vi "Get All Status Channels.vi"(8 "error in (no error)":errorcluster, 11 "VeriStand Data Sharing Framework in":refnum<class "VeriStand DSF.lvclass">) -> (0 "error out":errorcluster, 2 "status channel offsets":u64[](array[numeric]) format="%.0x", 3 "VeriStand Data Sharing Framework out":refnum<class "VeriStand DSF.lvclass">)   [LabVIEW 2017, in "DSF Engine.lvlib" / "VeriStand DSF.lvclass"]
uses:
  VeriStand DSF.lvclass
  VeriStand DSF.lvclass/VeriStand DSF.ctl
  <vilib>/NI Veristand/Custom Device API/Data Access Type.ctl
  <vilib>/NI Veristand/Custom Device API/Custom Device API.lvlib
  Shared/DSF Shared.lvlib
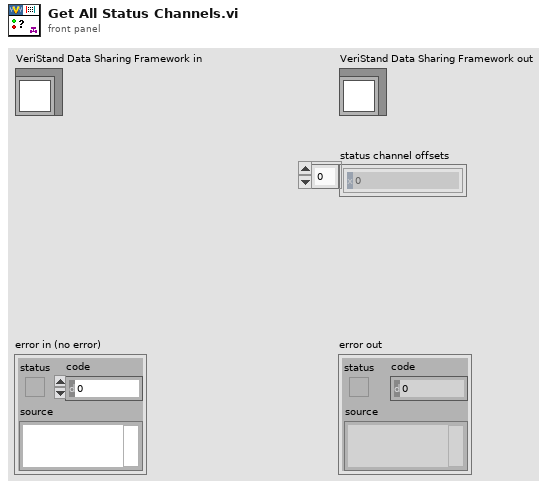
[diagram p1: front panel]
types:
  T1 = enum16{"open", "replace", "create", "open or create", "replace or create", "replace or create with confirmation"}
  T2 = typedef "Custom Device API.lvlib/Custom Device Item Ref.ctl" = u64
  T3 = typedef "Custom Device API.lvlib/Data Access Type.ctl" = enum16{"Read", "Write"}
  T4 = typedef "Custom Device API.lvlib/Data Reference.ctl" = i32
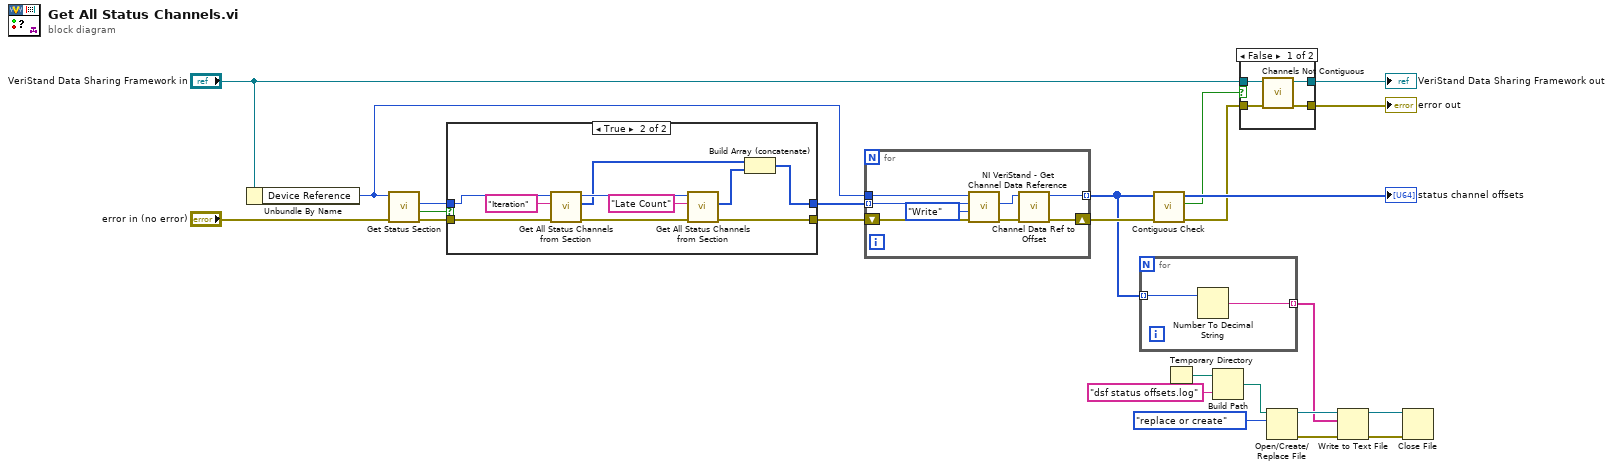
[diagram p0: block diagram]
diagram:
  n1 = Unbundle By Name("VeriStand Data Sharing Framework in") -> ("Device Reference"=w9:T2)
  n2 = call "Get Status Section.vi"("error in (no error)"="error in (no error)", "Item Ref in"=w9) -> ("error out"=w14:errorcluster, "found"=w2:bool, "Status Section ref"=w13:T2)  [unwired: 6 in, 1 out]
  n3 = case shown="True" w2 {
    tunnel: w14 -> [w25 w34]
    tunnel: w13 -> [_ w33]
    tunnel: [w25 w26] -> w12
    tunnel: [_ w35] -> w1
    frame False {
    }
    frame True {
      n4 = call "Get All Status Channels from Section.vi"("error in (no error)"=w34, "Section Name"="Iteration", "Item Ref in"=w33) -> ("error out"=w30:errorcluster, "status channels refs"=w28:T2[], "Item Ref out"=w31:T2)  [unwired: 6 in]
      n5 = call "Get All Status Channels from Section.vi"("error in (no error)"=w30, "Section Name"="Late Count", "Item Ref in"=w31) -> ("error out"=w26:errorcluster, "status channels refs"=w27:T2[])  [unwired: 6 in, 1 out]
      n6 = Build Array (concatenate)(w28, w27) -> (w35:T2[])
    }
  }
  n7 = for {
    shift-right: [w42] -> w11
    shift-left: w12 -> [w41]
    tunnel: [w39] -> w10 mode=indexing
    tunnel: w9 -> [w37]
    tunnel: w1 -> [w36] mode=indexing
    n8 = call <vilib>:"NI VeriStand - Get Channel Data Reference.vi"("error in (no error)"=w41, "Access"=Data_Access_Type."Write", "Channel Ref in"=w36, "Device Ref in"=w37) -> ("error out"=w43:errorcluster, "Channel Data Reference"=w40:T4)  [unwired: 5 in, 1 out]
    n9 = call "Channel Data Ref to Offset.vi"("error in (no error)"=w43, "Channel Data Reference"=w40) -> ("error out"=w42:errorcluster, "channel offset"=w39:u64)  [unwired: 8 in]
  }
  n10 = for {
    tunnel: [w45] -> w16 mode=indexing
    tunnel: w10 -> [w44] mode=indexing
    n11 = Number To Decimal String(number=w44) -> (decimal integer string=w45:string)  [unwired: 1 in]
  }
  n12 = call "Contiguous Check.vi"("error in (no error)"=w11, "channel offsets in"=w10) -> ("error out"=w4:errorcluster, "contiguous?"=w3:bool, "channel offsets out"=→"status channel offsets":u64[])  [unwired: 7 in]
  n13 = Temporary Directory() -> (w23:path)
  n14 = Build Path(base path=w23, name or relative path="dsf status offsets.log") -> (appended path=w21:path)
  n15 = case shown="False" w3 {
    tunnel: "VeriStand Data Sharing Framework in" -> [w49 w51]
    tunnel: [w48 w51] -> w7
    tunnel: [w47 w50] -> w6
    tunnel: w4 -> [w46 w50]
    frame False {
      n16 = call "Channels Not Contiguous.vi"("error in (no error)"=w46, "VeriStand DSF in"=w49) -> ("error out"=w47:errorcluster, "VeriStand DSF out"=w48:refnum<class "VeriStand DSF.lvclass">)  [unwired: 8 in]
    }
    frame True {
    }
  }
  "error out" <- w6
  "VeriStand Data Sharing Framework out" <- w7
  n17 = Open/Create/Replace File(file path (use dialog)=w21, operation (0:open)=T1."replace or create") -> (refnum out=w20:refnum<file>, error out=w19:errorcluster)  [unwired: 4 in, 1 out]
  n18 = Write to Text File(file (use dialog)=w20, text=w16, error in=w19) -> (refnum out=w17:refnum<file>, error out=w18:errorcluster)  [unwired: 1 in, 1 out]
  n19 = Close File(refnum=w17, error in=w18) -> ()  [unwired: 2 out]
